vi "Move Matrix.vi"(3 "Make Vertical":bool, 4 "Side":T2=enum."right", 5 "Label":string="Test", 6 "Wait Time":dbl, 8 "error in":errorcluster, 9 "Speed (mm/s)":dbl=50.0, 10 "Offset":T1 format="%.3f", 11 "Location":string) -> (0 "error out":errorcluster)   [LabVIEW 2013]
uses:
  ROS/Code/SubVIs/BaxterSide.ctl
  <vilib>/Analysis/Matrix/Datatypes/RealMatrix.ctl
  <vilib>/Analysis/Matrix/NI_Matrix.lvlib
panel:
  out "Final Offset":T1 format="%.3f"
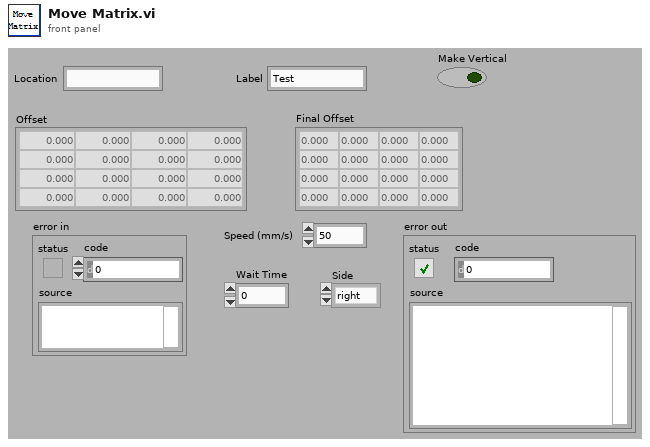
[diagram p1: front panel]
types:
  T1 = typedef "NI_Matrix.lvlib/RealMatrix.ctl" = dbl[][]
  T2 = typedef "BaxterSide.ctl" = enum16{"left", "right"}
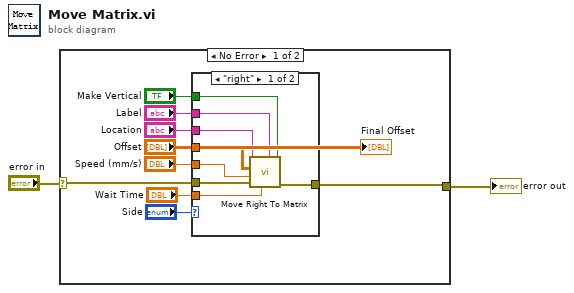
[diagram p0: block diagram]
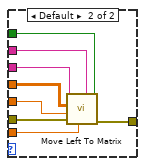
[diagram p2: hidden frame]
diagram:
  n1 = case shown="No Error" "error in" {
    selector: "error in" -> [w7 w28]
    tunnel: [w3 w28] -> w1
    frame No Error {
      n2 = case shown="\"right\"" "Side" {
        tunnel: "Make Vertical" -> [w19 w27]
        tunnel: "Label" -> [w18 w26]
        tunnel: "Location" -> [w17 w25]
        tunnel: "Offset" -> [w16 w24]
        tunnel: w7 -> [w15 w23]
        tunnel: "Speed (mm/s)" -> [w14 w22]
        tunnel: "Wait Time" -> [w13 w21]
        tunnel: [w12 w20] -> w3
        frame "right" {
          n3 = call "Move Right To Matrix.vi"("Make Vertical"=w19, "Label"=w18, "Wait Time"=w13, "error in"=w15, "Speed (mm/s)"=w14, "Goal Pose in Location"=w16, "Location"=w17) -> ("error out"=w12:errorcluster)  [unwired: 4 in]
        }
        frame Default {
          n4 = call "Move Left To Matrix.vi"("Make Vertical"=w27, "Label"=w26, "Wait Time"=w21, "error in"=w23, "Speed (mm/s)"=w22, "Offset"=w24, "Location"=w25) -> ("error out"=w20:errorcluster)  [unwired: 4 in]
        }
      }
      "Final Offset" <- "Offset"
    }
    frame Error {
    }
  }
  "error out" <- w1
